vi "Initialize.vi"(8 "error in (no error)":errorcluster, 9 "Reset (True)":bool=TRUE, 10 "ID Query (True)":bool=TRUE, 11 "VISA resource name":refnum<visa-resource-name>) -> (0 "error out":errorcluster, 3 "VISA resource name out":refnum<visa-resource-name>)   [LabVIEW 2020, in "ADCMT7451_ADC.lvlib"]
doc: "Establishes communication with the instrument and optionally performs an instrument identification query and/or an instrument reset. It also places the instrument in a default state needed for other instrument driver operations. Therefore, call this VI before calling other instrument driver VIs for this instrument. Generally, you need to call the Initialize VI only once at the beginning of an application."
uses:
  ADCMT7451_ADC.lvlib
  <vilib>/regexp/Match Regular Expression.xnode
panel:
  # "(c) 2008 ADC Corporation.  ALL RIGHTS RESERVED."
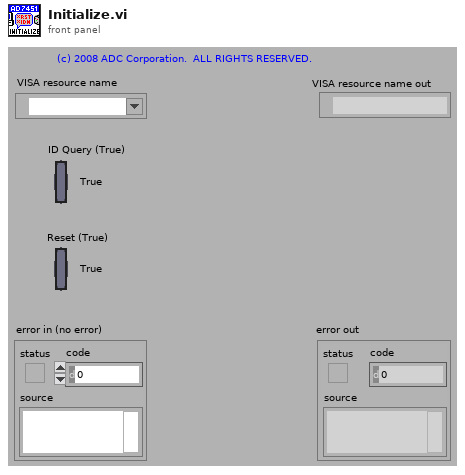
[diagram p1: front panel]
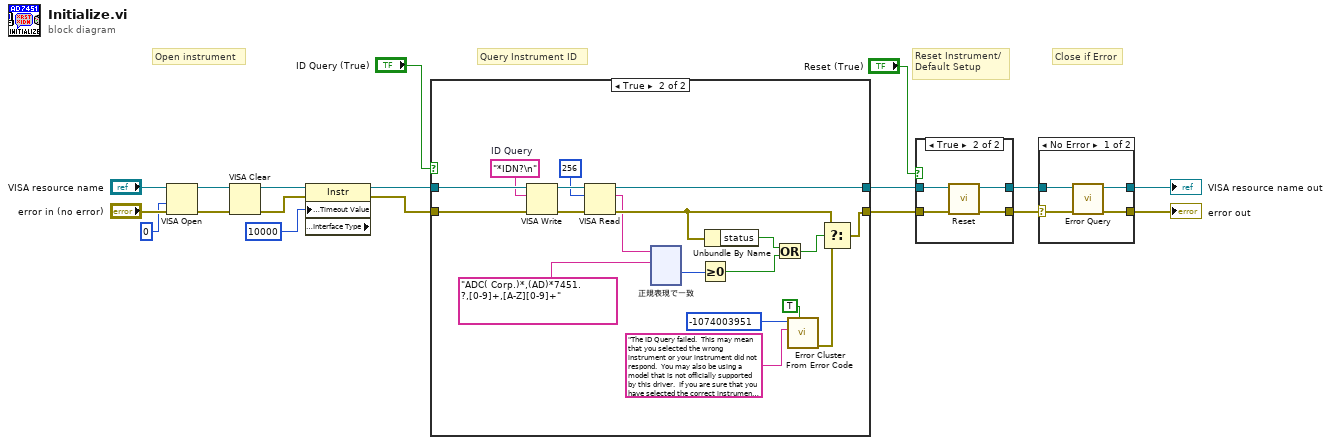
[diagram p0: block diagram]
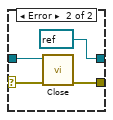
[diagram p2: hidden frame]
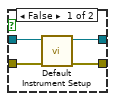
[diagram p3: hidden frame]
diagram:
  # "Close if Error"
  # "Query Instrument ID"
  # "Reset Instrument/\nDefault Setup"
  # "Open instrument"
  n1 = VISA Open(access mode=u32 0, error in (no error)="error in (no error)", VISA resource name="VISA resource name") -> (VISA resource name=w10:refnum<visa-resource-name>, error out=w9:errorcluster)  [unwired: 2 in]
  n2 = VISA Clear(VISA resource name=w10, error in (no error)=w9) -> (VISA resource name out=w8:refnum<visa-resource-name>, error out=w7:errorcluster)
  n3 = property class="Instr" props=["General Settings:Timeout Value", "Interface Information:Interface Type"](reference=w8, error in=w7, "General Settings:Timeout Value"=u32 10000) -> (reference out=w2:refnum<visa-resource-name>, error out=w1:errorcluster)  [unwired: 1 out]
  n4 = case shown="True" "ID Query (True)" {
    tunnel: [w19 w39] -> w17
    tunnel: [w20 w36] -> w18
    tunnel: w2 -> [w20 w37]
    tunnel: w1 -> [w19 w38]
    frame False {
    }
    frame True {
      w32 = "*IDN?\n"  # ID Query
      n5 = VISA Write(VISA resource name=w37, write buffer=w32, error in (no error)=w38) -> (VISA resource name out=w35:refnum<visa-resource-name>, error out=w34:errorcluster)  [unwired: 1 out]
      n6 = VISA Read(VISA resource name=w35, byte count=u32 256, error in (no error)=w34) -> (VISA resource name out=w36:refnum<visa-resource-name>, read buffer=w21:string, error out=w27:errorcluster)  [unwired: 1 out]
      n7 = xnode "正規表現で一致"("input string"=w21, "regular expression"="ADC( Corp.)*,(AD)*7451.?,[0-9]+,[A-Z][0-9]+") -> ("offset past match"=w22:i32)  [unwired: 4 in, 4 out]
      n8 = Greater Or Equal To 0?(x=w22) -> (x >= 0?=w25:bool)
      n9 = Unbundle By Name(w27) -> ("status"=w26:bool)
      n10 = Or(x=w26, y=w25) -> (x .or. y?=w24:bool)
      n11 = call <vilib>:"Error Cluster From Error Code.vi"("show call chain? (False)"=TRUE, "error message (\"\")"="The ID Query failed.  This may mean that you selected the wrong instrument or your instrument did not respond.  You may also be using a model that is not officially supported by this driver.  If you are sure that you have selected the correct instrument and it is responding, try disabling the ID Query." ("Source (VI Name)"), "error code (0)"=-1074003951 ("Code")) -> ("error out"=w31:errorcluster)  [unwired: 6 in]
      n12 = Select(t=w27, s=w24, f=w31) -> (s? t:f=w39:errorcluster)
    }
  }
  n13 = case shown="True" "Reset (True)" {
    tunnel: w17 -> [w156 w158]
    tunnel: [w155 w161] -> w3
    tunnel: w18 -> [w157 w159]
    tunnel: [w154 w160] -> w4
    frame False {
      n14 = call "Default Instrument Setup.vi"("error in (no error)"=w156, "VISA resource name"=w157) -> ("error out"=w155:errorcluster, "VISA resource name out"=w154:refnum<visa-resource-name>)  [unwired: 8 in]
    }
    frame True {
      n15 = call "Reset.vi"("error in (no error)"=w158, "VISA resource name"=w159) -> ("error out"=w161:errorcluster, "VISA resource name out"=w160:refnum<visa-resource-name>)  [unwired: 8 in]
    }
  }
  n16 = case shown="No Error" w3 {
    selector: w3 -> [w163 w167]
    tunnel: w4 -> [w162 w168]
    tunnel: [w165 refnum<visa-resource-name> refnum ("VISA resource name out")] -> w6
    tunnel: [w164 w169] -> w5
    frame No Error {
      n17 = call "Error Query.vi"("error in (no error)"=w163, "VISA resource name"=w162) -> ("error out"=w164:errorcluster, "VISA resource name out"=w165:refnum<visa-resource-name>)  [unwired: 6 in, 2 out]
    }
    frame Error {
      n18 = call "Close.vi"("error in (no error)"=w167, "VISA resource name"=w168) -> ("error out"=w169:errorcluster)  [unwired: 9 in]
    }
  }
  "VISA resource name out" <- w6
  "error out" <- w5
